vi "BenchSelector.vi"() -> ()   [LabVIEW 2019]
panel:
  out "Bench Selector":bool
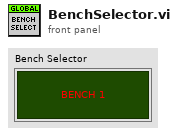
[diagram p1: front panel]
diagram:
